vi "filter.vi"(8 "deBaseline":bool, 9 "right rank":i32=-1, 10 "left rank":i32=2, 11 "data":dbl[](array[numeric])) -> (3 "filtered data":dbl[](array[numeric]))   [LabVIEW 2013]
uses:
  <vilib>/Analysis/2dsp.llb/1D Convolution (DBL).vi
  <vilib>/Analysis/NI_AALPro.lvlib
  <vilib>/Analysis/NI_AALBase.lvlib
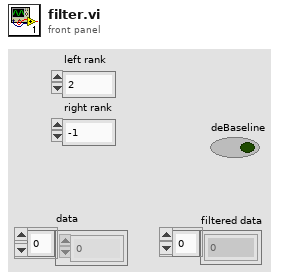
[diagram p1: front panel]
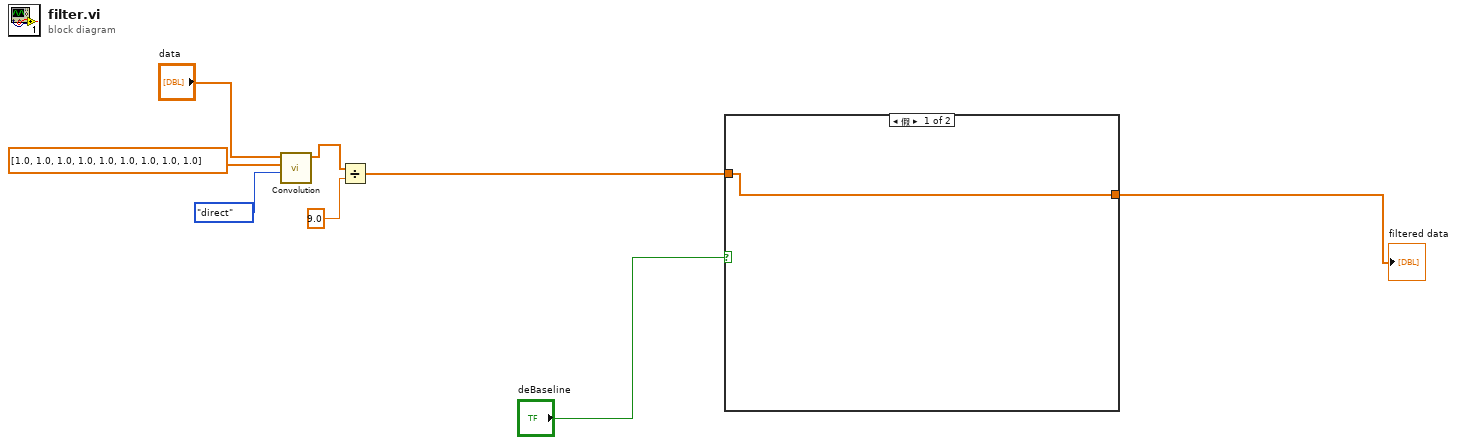
[diagram p0: block diagram]
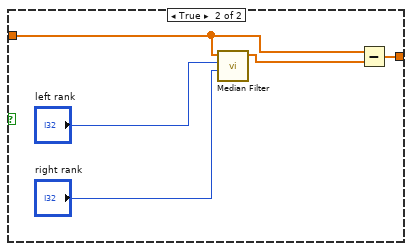
[diagram p2: hidden frame]
diagram:
  n1 = call-poly <vilib>:"Convolution.vi"("algorithm"=enum32{"direct", "frequency domain"}."direct", "Y"=dbl[] [1.0, 1.0, 1.0, 1.0, 1.0, 1.0, 1.0, 1.0, 1.0], "X"="data") -> ("X * Y"=w6:dbl[])  [unwired: 7 in, 1 out]
  n2 = Divide(x=w6, y=9.0) -> (x/y=w2:dbl[])
  n3 = case shown="假" "deBaseline" {
    tunnel: w2 -> [w9 w11]
    tunnel: [w9 w10] -> w1
    frame False {
    }
    frame True {
      n4 = call <vilib>:"Median Filter.vi"("right rank"="right rank", "left rank"="left rank", "X"=w11) -> ("Filtered X"=w14:dbl[])  [unwired: 7 in, 1 out]
      n5 = Subtract(x=w11, y=w14) -> (x-y=w10:dbl[])
    }
  }
  "filtered data" <- w1
